vi "KB-对角线消杂讯.vi"(10 "对角线高度值":dbl[](array[numeric]), 11 "外环3D":dbl[][](array[numeric])) -> (3 "消杂讯数据":dbl[][](array[numeric]))   [LabVIEW 2015]
panel:
  out "x/y":dbl
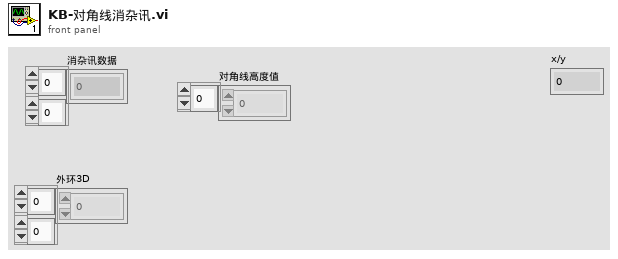
[diagram p1: front panel]
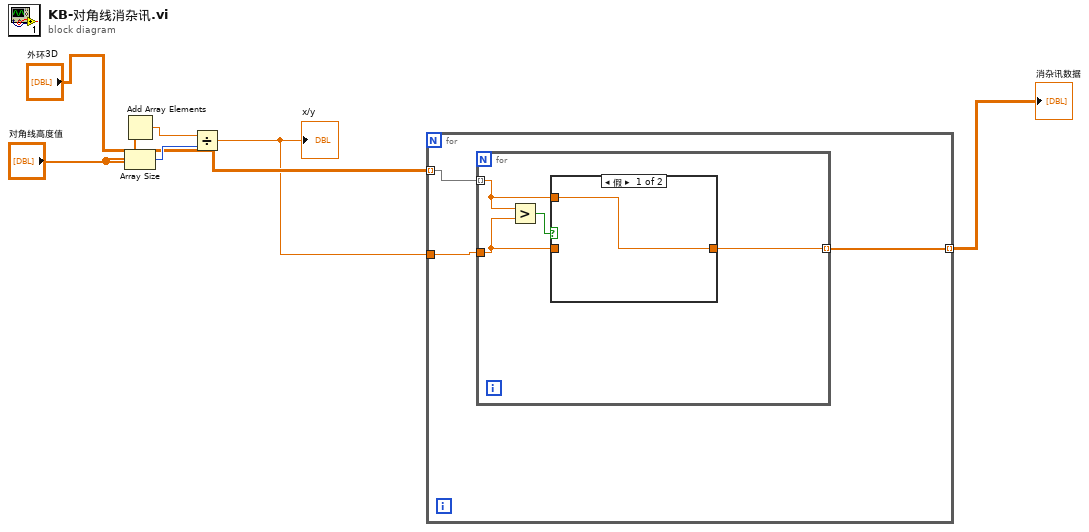
[diagram p0: block diagram]
diagram:
  n1 = Add Array Elements(numeric array="对角线高度值") -> (sum=w5:dbl)
  n2 = Array Size(array="对角线高度值") -> (size(s)=w4:i32)
  n3 = Divide(x=w5, y=w4) -> (x/y=w2:dbl)
  "x/y" <- w2
  n4 = for {
    tunnel: "外环3D" -> [w9] mode=indexing
    tunnel: w2 -> [w8]
    tunnel: [w7] -> w1 mode=indexing
    n5 = for {
      tunnel: w9 -> [w11] mode=indexing
      tunnel: w8 -> [w12]
      tunnel: [w10] -> w7 mode=indexing
      n6 = Greater?(x=w11, y=w12) -> (0:w13:bool)
      n7 = case shown="假" w13 {
        tunnel: [w14 w15] -> w10
        tunnel: w12 -> [_ w15]
        tunnel: w11 -> [w14 _]
        frame False {
        }
        frame True {
        }
      }
    }
  }
  "消杂讯数据" <- w1
